vi "Handle Request.vi"(7 "Arguments In":refnum<class "Arguments.lvclass">, 8 "error in (no error)":errorcluster, 10 "Request In":refnum<class "Request.lvclass">, 11 "TestQueryAuth in":refnum<class "TestQueryAuth.lvclass">) -> (0 "error out":errorcluster, 1 "Early Response":refnum<class "Response.lvclass">, 2 "Request":refnum<class "Request.lvclass">, 5 "Arguments":refnum<class "Arguments.lvclass">)   [LabVIEW 2020, in "TestQueryAuth.lvclass"]
uses:
  TestQueryAuth.lvclass
  HTTP Server/Arguments/Arguments.lvclass
  <vilib>/IlluminatedG/IG HTTP Utils/HTTP Utils/Request/Request.lvclass
  <vilib>/IlluminatedG/IG HTTP Utils/HTTP Utils/Response/Response.lvclass
  HTTP Server/Redirect Response/Redirect Response.lvclass
  C:/Program Files (x86)/National Instruments/LabVIEW 2020/vi.lib/IlluminatedG/IG HTTP Utils/HTTP Utils/Response/Response.lvclass
  TestQueryAuth.lvclass/TestQueryAuth.ctl
  <vilib>/IlluminatedG/lv-stream/URI/URI.lvclass
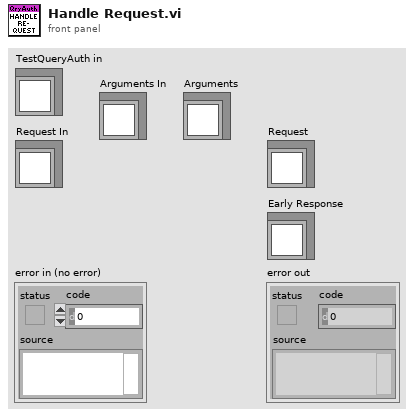
[diagram p1: front panel]
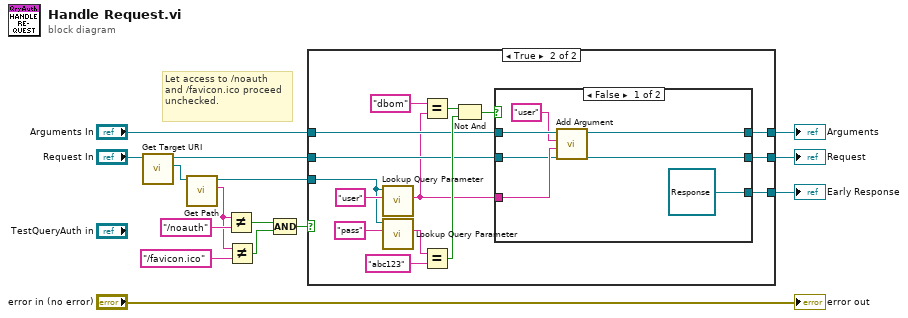
[diagram p0: block diagram]
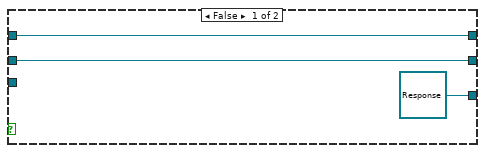
[diagram p2: hidden frame]
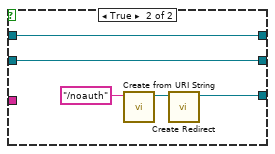
[diagram p3: hidden frame]
diagram:
  # "Let access to /noauth and /favicon.ico proceed unchecked."
  n1 = call <vilib>:"Get Target URI.vi"("Request in"="Request In") -> ("Target URI"=w8:refnum<class "URI.lvclass">, "Request out"=w11:refnum<class "Request.lvclass">)  [unwired: 8 in, 1 out]
  n2 = call <vilib>:"Get Path.vi"("URI in"=w8) -> ("Path"=w4:string, "URI out"=w6:refnum<class "URI.lvclass">)  [unwired: 8 in, 1 out]
  n3 = Not Equal?(x=w4, y="/noauth") -> (x != y?=w3:bool)
  n4 = Not Equal?(x=w4, y="/favicon.ico") -> (x != y?=w2:bool)
  n5 = Compound Arithmetic op=AND(w3, w2) -> (w1:bool)
  n6 = case shown="True" w1 {
    tunnel: "Arguments In" -> [w18 w25]
    tunnel: [w18 w24] -> w12
    tunnel: w11 -> [w17 w23]
    tunnel: [w17 w22] -> w10
    tunnel: [refnum<class "Response.lvclass"> refnum ("Early Response") w20] -> w9
    tunnel: w6 -> [_ w19]
    frame False {
    }
    frame True {
      n7 = call <vilib>:"Lookup Query Parameter.vi"("Name"="user", "URI in"=w19) -> ("Value"=w21:string)  [unwired: 6 in, 3 out]
      n8 = call <vilib>:"Lookup Query Parameter.vi"("Name"="pass", "URI in"=w19) -> ("Value"=w31:string)  [unwired: 6 in, 3 out]
      n9 = Equal?(x="dbom" ("y"), y=w21) -> (x = y?=w28:bool)
      n10 = Equal?(x=w31, y="abc123") -> (x = y?=w27:bool)
      n11 = Not And(1:w27, 2:w28) -> (0:w26:bool)
      n12 = case shown="False" w26 {
        tunnel: w25 -> [w39 w44]
        tunnel: [w36 w44] -> w24
        tunnel: w23 -> [w35 w43]
        tunnel: [w35 w43] -> w22
        tunnel: w21 -> [w38 _]
        tunnel: [refnum<class "Response.lvclass"> refnum ("Early Response") w40] -> w20
        frame False {
          n13 = call "Add Argument.vi"("Value"=w38, "Name"="user", "Arguments in"=w39) -> ("Arguments out"=w36:refnum<class "Arguments.lvclass">)  [unwired: 7 in, 1 out]
        }
        frame True {
          n14 = call <vilib>:"Create from URI String.vi"("URI String"="/noauth") -> ("URI out"=w42:refnum<class "URI.lvclass">)  [unwired: 9 in, 1 out]
          n15 = call "Create Redirect.vi"("Redirect URI"=w42) -> ("Redirect Response out"=w40:refnum<class "Redirect Response.lvclass">)  [unwired: 9 in, 1 out]
        }
      }
    }
  }
  "Arguments" <- w12
  "Request" <- w10
  "Early Response" <- w9
  "error out" <- "error in (no error)"
